vi "RunTest.vi"(8 "error in (no error)":errorcluster, 11 "AjustesPrevios in":refnum<class "AjustesPrevios.lvclass">) -> (0 "error out":errorcluster, 2 "resultado":string, 3 "AjustesPrevios out":refnum<class "AjustesPrevios.lvclass">)   [LabVIEW 2019, in "AjustesPrevios.lvclass"]
uses:
  AjustesPrevios.lvclass
  Prueba04/Control/Slide.ctl
  Controles/MessageAjustesPrev.ctl
  Controles/EstadosAjsutesPrev.ctl
  AjustesPrevios.lvclass/AjustesPrevios.ctl
  QMH/Message Queue/Enqueue Message (Single).vi
  RerenceAllControlsToolkit/_get control reference by name.vi
  RerenceAllControlsToolkit/_get mutiple control reference by name.vi
  Globals/globales.vi
  <vilib>/Utility/miscctls.llb/LVRowAndColumnTypeDef.ctl
  Prueba/Prueba.lvclass
  QMH/User Event - Stop/User Event - Stop.lvlib
  QMH/Message Queue/Message Queue.lvlib
  Prueba04/Prueba04.lvclass
panel:
  out "Sim":bool
  out "Vguardado":dbl
  out "size_frec":i32
  in  "Tabs":enum32{"Ajustes 1", "Ajustes 2", "Ajustes 3"}(tab)
  out "factor_correccion_enviado":dbl format="%#.5g"
  in  "aplicar FC":bool
  out "Voltaje mV":dbl format="%#.3g"
  out "Nivel Medido":dbl format="%#.2g"
  out "temperatura":dbl
  out "presion":dbl
  in  "humedad":dbl
  out "nivel_emitido":dbl
  out "factor_correccion":dbl format="%#.5g"
  in  "siguiente1":bool
  in  "Sensibilidad":dbl(knob)=0.1 scale=0.01..1.0 scale format="%#_6p"
  out "voltaje a CAM":dbl format="%.1f"
  out "frecuencia":dbl
  in  "guardar":bool
  in  "generar":bool
  in  "anterior2":bool
  in  "ajusteAmp(mV)":T1=1.0 caption="Ajuste de amplitud [V]" scale=0.1..1.5
  in  "siguiente2":bool
  in  "generar_CAM":bool
  out "voltaje":dbl format="%_3g"
  out "frecuencia":dbl
  out "NPS":dbl format="%#_4g"
  in  "anterior3":bool
  in  "terminar":bool
  out "Tabla":string[][](table)
  # "Información Pistófono"
  # "Nivel Medido [dB]"
  # "Factor de Corrección Calculado"
  # "Factor de Corrección Enviado"
  # "Voltaje [V]"
  # "Temperatura [°C]"
  # "Presión [hPa]"
  # "Humedad [%]"
  # "Nivel Emitido [dB]"
  # "Ajuste Previo 1 : Igualación de Patrones"
  # "Monitoreo"
  # "Voltaje a CAM"
  # "V"
  # "Frecuencia"
  # "Hz"
  # "Ajuste Previo 2 : Ajuste Acústico Emisor Multitono"
  # "Monitoreo"
  # "NPS"
  # "dB"
  # "Voltaje a CAM"
  # "V"
  # "Frecuencia"
  # "Hz"
  # "Ajuste Previo 3 : Niveles de Presión Sonora de Referencia"
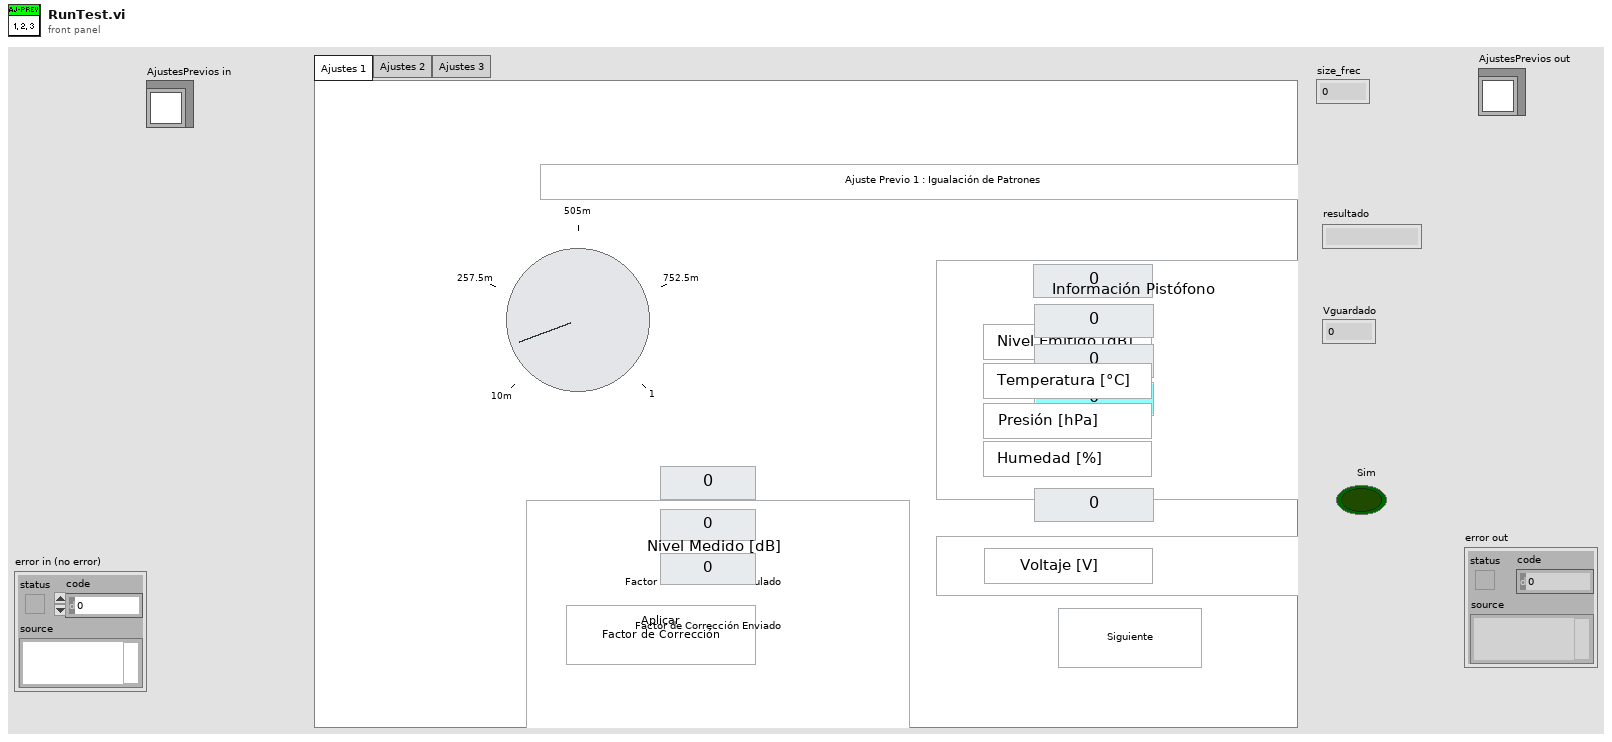
[diagram p1: front panel]
types:
  T1 = typedef "Prueba04.lvclass/Slide.ctl" = dbl
  T2 = typedef "Prueba.lvclass/MessageAjustesPrev.ctl" = cluster{"Estados":T3, "Data":variant}
  T3 = typedef "Prueba.lvclass/EstadosAjsutesPrev.ctl" = enum16{"inicio", "iniciaInstrumentos", "configurarTabla", "Ajustes1", "escribeSensib", "aplicarFC", "escribir_datos_igual_patrones", "preguntar_gen", "Ajustes2", "generar", "detenerGEN", "monitorear", "guardar", "Ajustes3", "generarCAM_94", "avisoParaCAM114", "generarCAM_114", "salir", "error", "reconec_pistofono"}
  T4 = typedef "LVRowAndColumnTypeDef.ctl" = cluster{"Row":i32, "Column":i32}
  T5 = typedef "Message Queue.lvlib/All Message Queues.ctl" = cluster{"MHL":refnum<queue>, "Inst_CNT90":refnum<queue>, "Inst_DS360":refnum<queue>, "Inst_Keithley2002":refnum<queue>, "Inst_DAQ":refnum<queue>, "BD":refnum<queue>, "Pistofono":refnum<queue>, "Nexus":refnum<queue>}
  T6 = enum8{"Enabled", "Disabled", "Disabled and Grayed Out"}
  T7 = cluster{"ControlName":string, "ControlReference":refnum<vi>}[]
  T8 = cluster{"Nivel Emitido Pistófono [dB]":dbl, "Temperatura interna Pistófono[ºC]":dbl, "Presión Medida Pistófono  [hPa]":dbl, "Humedad Relativa Aire [%]":dbl, "FactorCorreccionSensNexus":dbl}
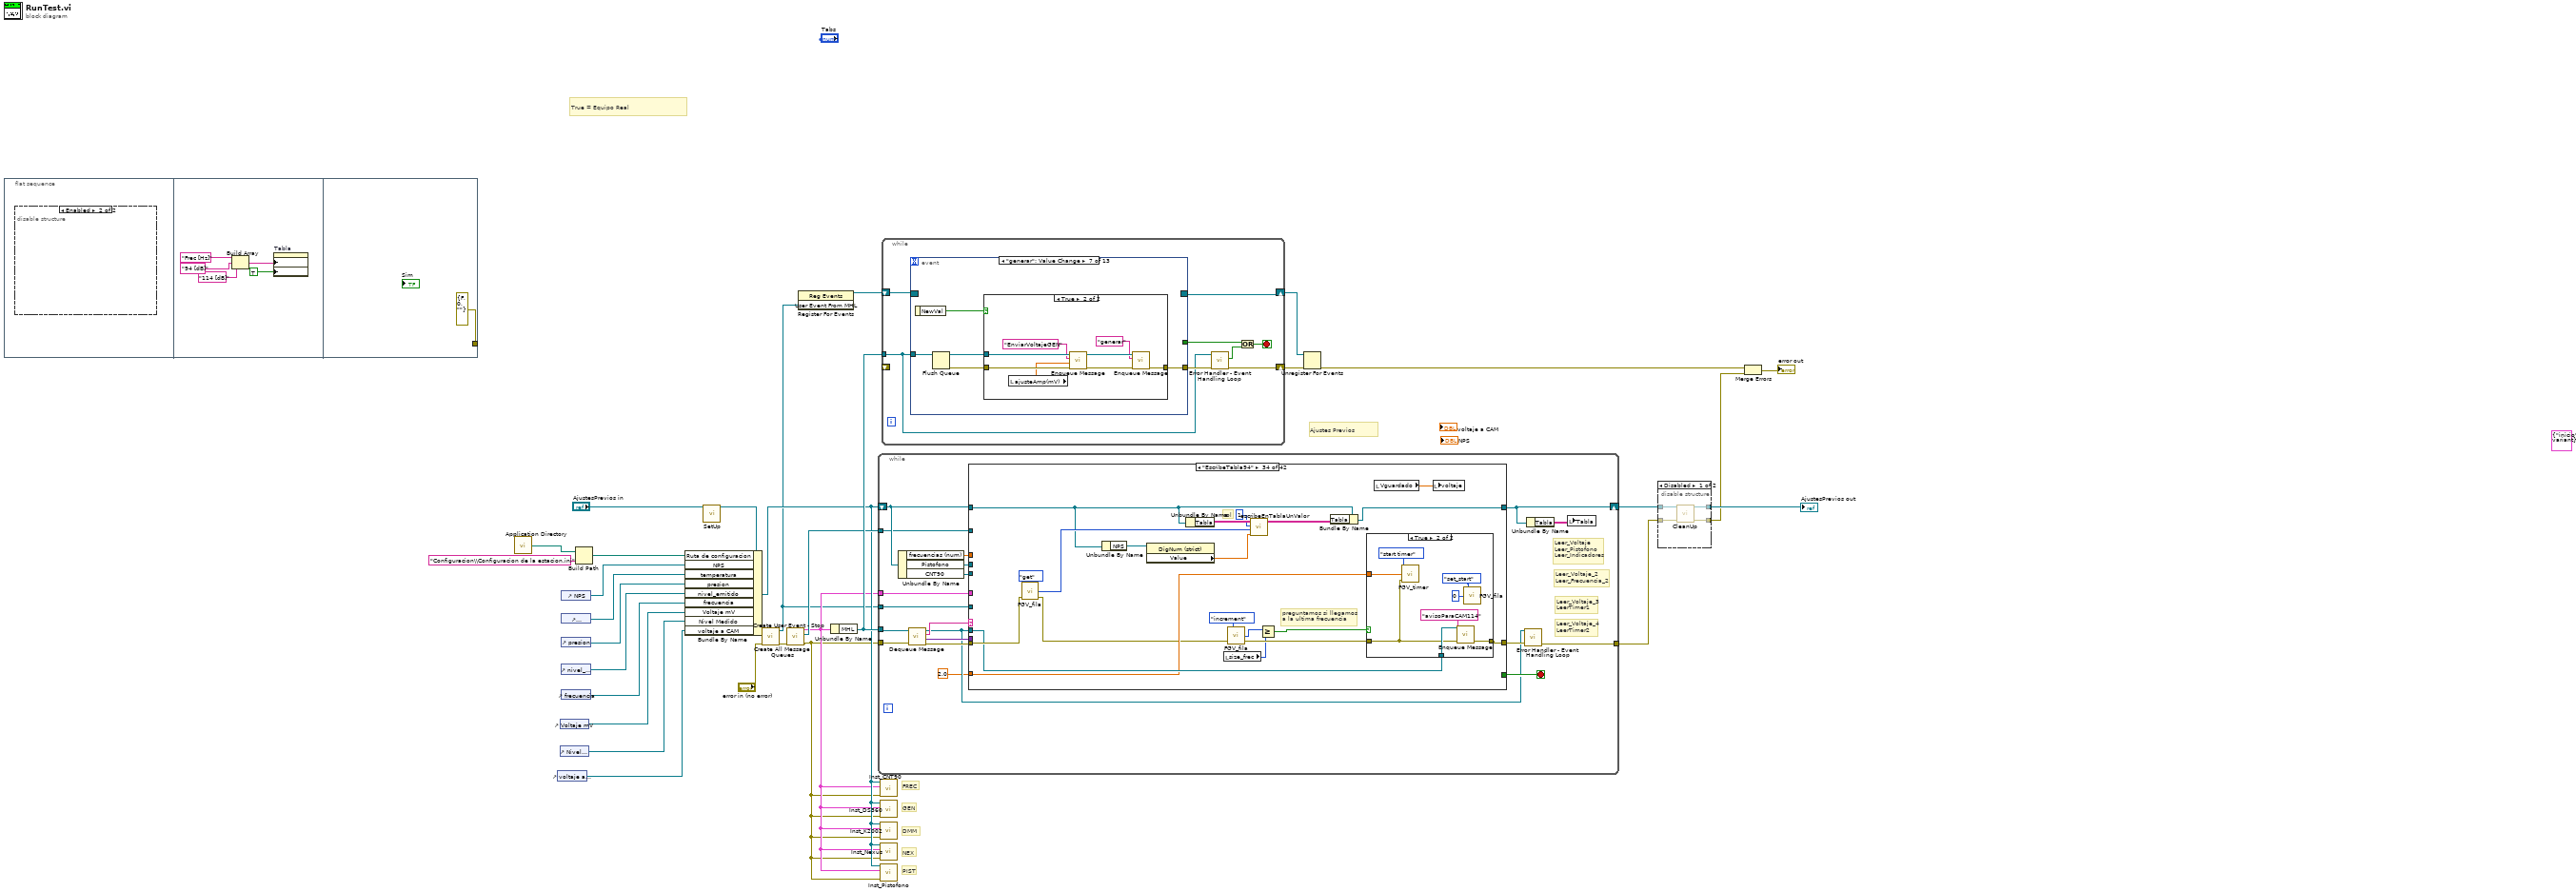
[diagram p0: block diagram]
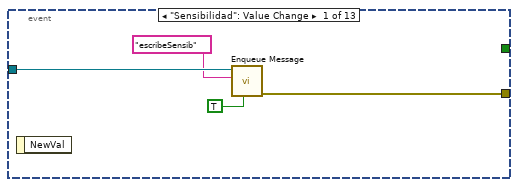
[diagram p3: hidden frame]
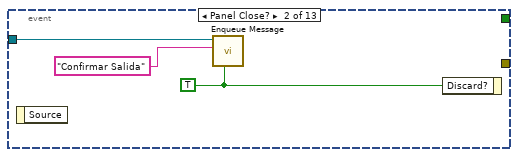
[diagram p4: hidden frame]
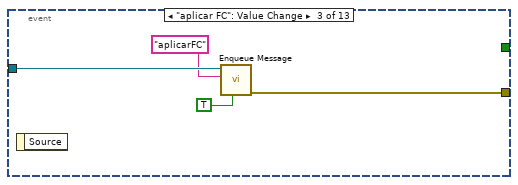
[diagram p5: hidden frame]
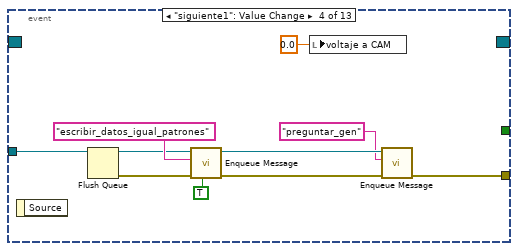
[diagram p6: hidden frame]
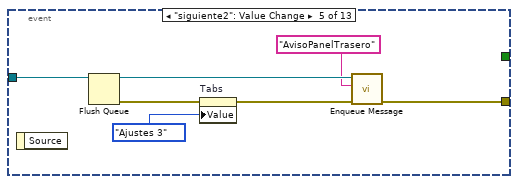
[diagram p7: hidden frame]
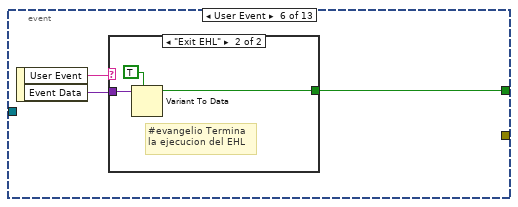
[diagram p8: hidden frame]
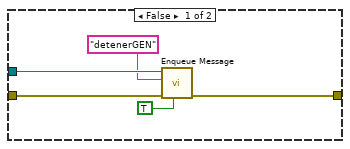
[diagram p10: hidden frame]
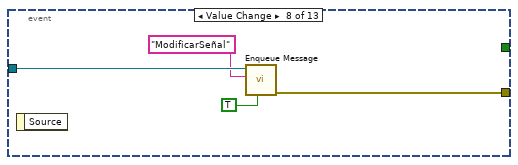
[diagram p11: hidden frame]
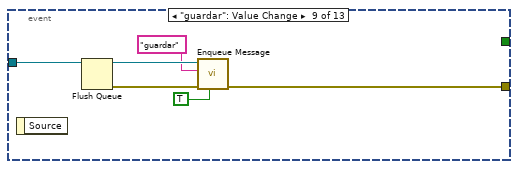
[diagram p12: hidden frame]
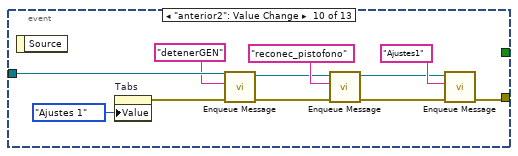
[diagram p13: hidden frame]
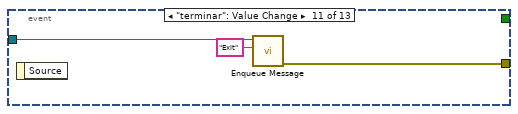
[diagram p14: hidden frame]
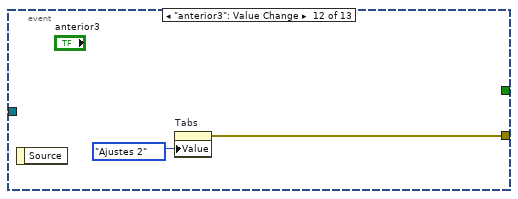
[diagram p15: hidden frame]
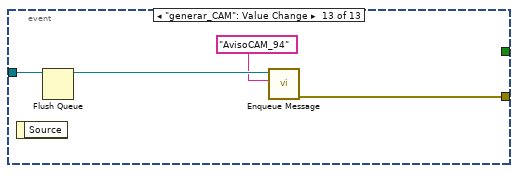
[diagram p16: hidden frame]
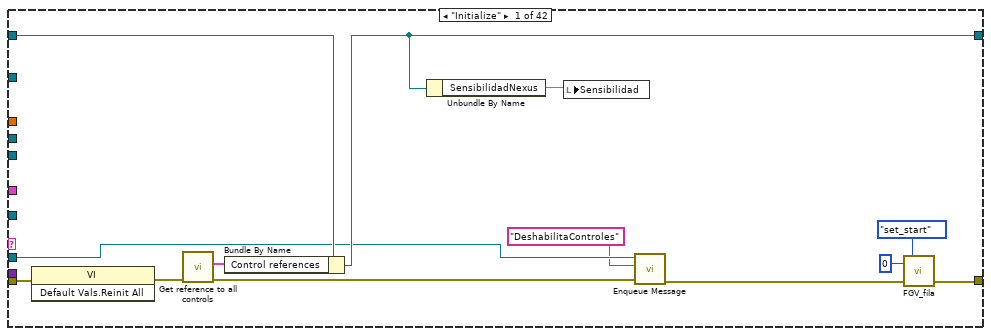
[diagram p17: hidden frame]
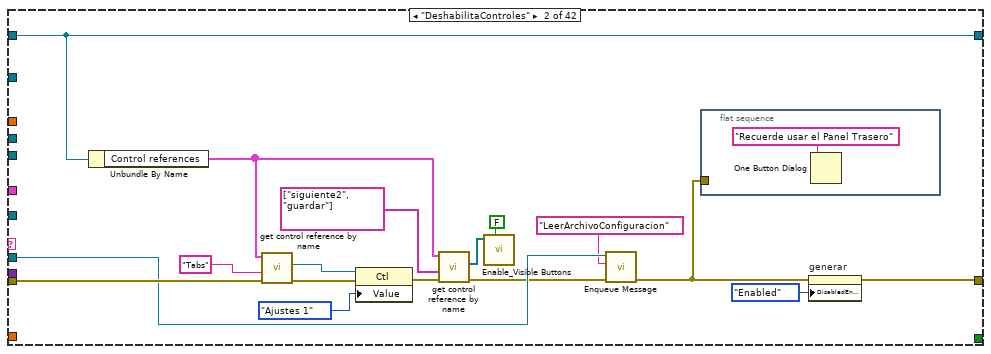
[diagram p18: hidden frame]
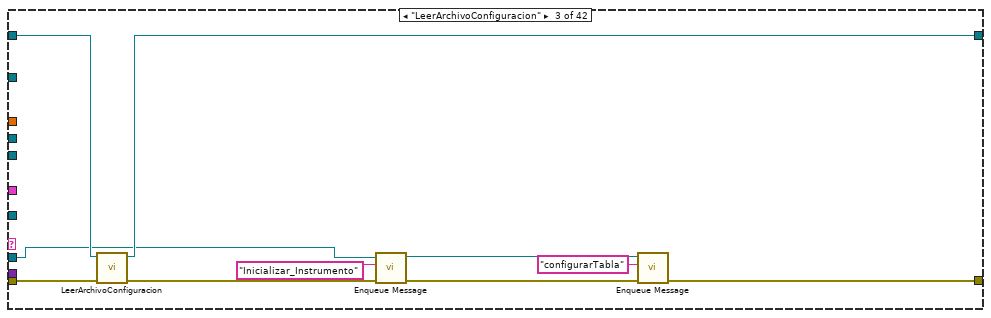
[diagram p19: hidden frame]
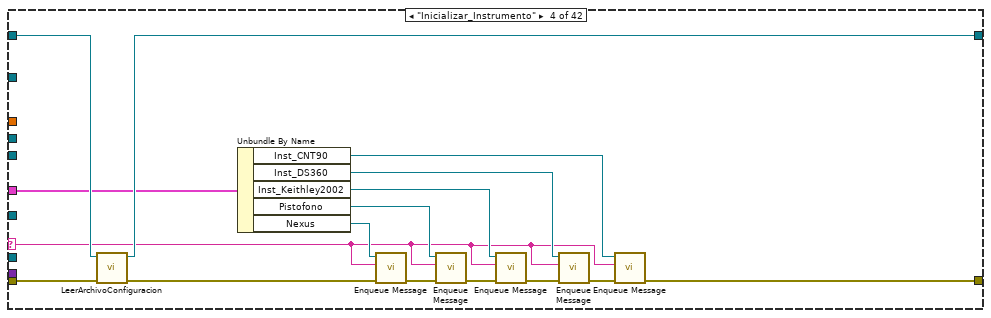
[diagram p20: hidden frame]
diagram:
  (unwired) T2 {"Estados"=enum."inicio", "Data"=variant}
  # "PIST"
  # "NEX"
  # "FREC"
  # "GEN"
  # "DMM"
  # "Ajustes Previos"
  # "True = Equipo Real"
  n1 = flat-sequence {
    tunnel: [errorcluster {"status"=FALSE, "code"=0, "source"=""} ("error in (no error)")] -> _
    frame #0 {
      n2 = disable-structure shown="Enabled" {
        frame Disabled {
          n3 = Bundle By Name(cluster=T4 {"Row"=0, "Column"=0} ("Active Cell:Active Cell"), "Row"=-2, "Column"=-2) -> (w36:T4)
          n4 = property on="Tabla" class="Tbl (strict)"("Active Cell"=w36, "CellFontSize"=u32 20 ("Active Cell:Cell Font:Size"), "Justify"=enum16{"Left", "Center", "Right"}."Center" ("Active Cell:Cell Justification")) -> ()  [unwired: 2 in, 2 out]
        }
        frame Enabled {
        }
      }
    }
    frame #1 {
      n5 = Build Array("Frec [Hz]", "94 [dB]", "114 [dB]" ("element")) -> (w38:string[])
      n6 = property on="Tabla" class="Tbl (strict)"("Column Headers[]"=w38, "Col Headers Vis"=TRUE ("Visible Items:Column Headers Visible")) -> ()  [unwired: 2 in, 2 out]
    }
    frame #2 {
    }
  }
  n7 = call <vilib>:"Application Directory.vi"() -> ("Application Directory"=w20:path)
  n8 = control-ref of="voltaje a CAM"() -> (w1:refnum<vi>)
  n9 = control-ref of="Voltaje mV"() -> (w3:refnum<vi>)
  n10 = control-ref of="Nivel Medido"() -> (w2:refnum<vi>)
  n11 = control-ref of="NPS"() -> (w8:refnum<vi>)
  n12 = control-ref of="temperatura"() -> (w7:refnum<vi>)
  n13 = control-ref of="presion"() -> (w6:refnum<vi>)
  n14 = control-ref of="nivel_emitido"() -> (w5:refnum<vi>)
  n15 = control-ref of="frecuencia"() -> (w4:refnum<vi>)
  n16 = Build Path(base path=w20, name or relative path="Configuracion\\Configuracion de la estacion.ini") -> (appended path=w19:path)
  n17 = call-dynamic "SetUp.vi"("AjustesPrevios in"="AjustesPrevios in") -> ("AjustesPrevios out"=w18:refnum<class "AjustesPrevios.lvclass">)  [unwired: 9 in, 1 out]
  n18 = Bundle By Name(cluster=w18, "Ruta de configuracion"=w19, "NPS"=w8, "temperatura"=w7, "presion"=w6, "nivel_emitido"=w5, "frecuencia"=w4, "Voltaje mV"=w3, "Nivel Medido"=w2, "voltaje a CAM"=w1) -> (w14:refnum<class "AjustesPrevios.lvclass">)
  n19 = call "Create User Event - Stop.vi"("error in (no error)"="error in (no error)") -> ("error out"=w22:errorcluster, "User Event From MHL"=w12:refnum<user-event>)  [unwired: 9 in]
  n20 = call "Create All Message Queues.vi"("error in (no error)"=w22) -> ("error out"=w9:errorcluster, "PL Queues Array"=w15:refnum<queue>[], "All Message Queues out"=w13:T5)  [unwired: 8 in]
  n21 = register-events(w12) -> (reference out=w26:refnum<event-registration>)  [unwired: 2 in, 1 out]
  n22 = Unbundle By Name(w13) -> ("MHL"=w16:refnum<queue>)
  n23 = while {
    tunnel: w16 -> [w54]
    tunnel: w9 -> [w53]
    shift-right: [w59] -> w27
    shift-left: w14 -> [w60]
    tunnel: w13 -> [w49]
    tunnel: w15 -> [w48]
    tunnel: w12 -> [w47]
    tunnel: [w44] -> w11
    stop <- w61 stop-if-true
    # "Leer_Voltaje_4\nLeerTimer2"
    # "Leer_Voltaje_3\nLeerTimer1"
    # "Leer_Voltaje_2\nLeer_Frecuencia_2"
    # "Leer_Voltaje\nLeer_Pistofono\nLeer_Indicadores"
    n24 = Unbundle By Name(w60) -> ("frecuencias (num)"=w56:dbl[], "Pistofono"=w57:refnum<class "Pistofono.lvclass">, "CNT90"=w55:refnum<class "CNT90.lvclass">)
    n25 = call "Dequeue Message.vi"("error in (no error)"=w53, "Message Queue"=w54) -> ("error out"=w52:errorcluster, "Message Data"=w50:variant, "Message"=w51:string, "dup Message Queue"=w45:refnum<queue>)  [unwired: 6 in]
    n26 = case shown="\"EscribeTabla94\"" w51 {
      selector: w51 -> [_ _ _ w103 _ w129 _ _ _ _ _ _ _ _ _ _ _ _ _ _ _ _ _ _ _ _ _ _ _ _ _ _ _ _ _ _ _ _ w570 _ _ _]
      tunnel: w52 -> [w69 w90 w101 w117 w127 w141 w153 w156 w173 w184 w195 w206 w222 w234 w239 w245 w265 w280 w284 w299 w317 w328 w334 w349 w359 w367 w369 w378 w388 w397 w416 w423 w435 w468 w493 w503 w515 w536 w573 w590 w595 w597]
      tunnel: [w74 w76 w97 w102 w121 w128 w143 w155 w173 w174 w185 w196 w210 w229 w238 w247 w266 w280 w281 w295 w307 w318 w330 w344 w350 w365 w369 w378 w385 w396 w405 w421 w441 w466 w487 w498 w513 w545 w566 w584 w595 w597] -> w46
      tunnel: [_ _ _ _ _ _ _ _ _ _ _ _ _ _ _ _ _ _ _ _ _ _ _ _ _ _ _ _ _ _ _ _ _ _ _ _ _ _ w568 _ _ _] -> w61
      tunnel: w60 -> [w67 w91 w99 w115 w124 w140 w152 w162 w172 w183 w194 w205 w217 w232 w243 w250 w259 w279 w293 w306 w316 w327 w340 w345 w358 w366 w368 w377 w382 w398 w418 w432 w450 w453 w492 w512 w529 w532 w569 w593 w594 w596]
      tunnel: [w66 w91 w98 w114 w122 w140 w152 w162 w172 w183 w194 w205 w219 w233 w244 w257 w258 w279 w293 w306 w316 w327 w340 w345 w356 w366 w368 w375 w382 w398 w418 w432 w450 w460 w492 w512 w529 w540 w569 w593 w594 w596] -> w59
      tunnel: w57 -> [_ _ _ _ _ _ _ _ _ _ _ _ _ _ _ _ _ _ _ _ _ _ _ _ _ _ _ _ _ _ _ _ _ _ _ _ _ _ _ _ _ _]
      tunnel: w56 -> [_ _ _ _ _ _ _ _ _ _ _ _ _ _ _ _ _ _ _ _ _ _ _ _ _ _ _ _ _ _ _ _ w436 _ _ _ w517 _ _ _ _ _]
      tunnel: w55 -> [_ _ _ _ _ _ _ _ _ _ _ _ _ _ _ _ _ _ _ _ _ _ _ _ _ _ _ _ _ _ _ _ _ _ _ _ _ _ _ _ _ _]
      tunnel: w45 -> [w65 w80 w96 _ w119 _ _ w157 _ w182 w193 w204 w212 _ _ _ w263 _ _ w296 w315 w326 w333 _ w354 _ _ _ w386 w395 w409 w420 w443 w458 w491 w502 w514 w537 w572 w586 _ _]
      tunnel: w50 -> [_ _ _ _ _ _ _ _ _ _ _ _ _ _ _ _ _ _ w283 _ _ _ _ _ _ _ _ _ _ _ _ _ _ _ _ _ _ _ _ w589 _ _]
      tunnel: w49 -> [_ _ _ w113 _ w139 w151 _ _ w180 w191 w202 _ w228 w242 w249 _ _ w282 w298 w313 w324 w332 w348 _ w364 _ _ w387 _ w415 w422 _ _ _ w501 _ _ _ _ _ _]
      tunnel: w48 -> [_ _ _ _ _ _ _ _ _ _ _ _ _ _ _ _ _ _ _ _ _ _ _ _ _ _ _ _ _ _ _ _ _ _ _ _ _ _ w567 _ _ _]
      tunnel: w47 -> [_ _ _ _ _ _ _ _ _ _ _ _ _ _ _ _ _ _ _ _ _ _ _ _ _ _ _ _ _ _ _ _ _ _ _ _ _ _ w571 _ _ _]
      tunnel: 2.0 ("time target") -> [_ _ _ _ _ _ _ _ _ _ _ _ _ _ _ _ _ _ _ _ _ _ _ _ _ _ _ _ _ _ w402 _ _ w455 w485 _ _ w533 _ _ _ _]
      frame "Initialize" {
        n27 = invoke class="VI" method="Default Vals.Reinit All"(error in=w69) -> (error out=w70:errorcluster)  [unwired: 2 in, 2 out]
        n28 = call "Get reference to all controls.vi"("error in (no error)"=w70) -> ("error out"=w63:errorcluster, "Control references"=w68:T7)  [unwired: 5 in]
        n29 = Bundle By Name(cluster=w67, "Control references"=w68) -> (w66:refnum<class "AjustesPrevios.lvclass">)
        n30 = Unbundle By Name(w66) -> ("SensibilidadNexus"=w71:dbl)
        n31 = local write "Sensibilidad"(w71) -> ()
        n32 = call-poly "Enqueue Message.vi"("error in (no error)"=w63, "Message"="DeshabilitaControles", "Message Queue"=w65) -> ("error out"=w62:errorcluster)  [unwired: 7 in, 1 out]
        n33 = call "FGV_fila.vi"("error in (no error)"=w62, "fila_inicial"=0, "action"=enum16{"increment", "set_start", "get"}."set_start") -> ("error out"=w74:errorcluster)  [unwired: 1 in, 1 out]
      }
      frame "DeshabilitaControles" {
        n34 = Unbundle By Name(w91) -> ("Control references"=w81:T7)
        n35 = call-poly "get control reference by name.vi"("error in (no error)"=w90, "Control name"="Tabs", "Control references"=w81) -> ("error out"=w88:errorcluster, "Ctl Refnum"=w85:refnum<vi>)  [unwired: 3 in]
        n36 = property on="Property Node" class="Ctl"(reference=w85, error in=w88, "Value"=enum32{"Ajustes 1", "Ajustes 2", "Ajustes 3"}."Ajustes 1" ("Tabs")) -> (error out=w87:errorcluster)  [unwired: 1 out]
        n37 = call-poly "get control reference by name.vi"("error in (no error)"=w87, "Control names"=string[] ["siguiente2", "guardar"] ("Control name"), "Control references"=w81) -> ("error out"=w79:errorcluster, "References"=w82:refnum<vi>[])  [unwired: 3 in]
        n38 = call "Enable_Visible Buttons.vi"("Enable? (T)"=FALSE, "Controls Ref Array"=w82) -> ()  [unwired: 10 in]
        n39 = call-poly "Enqueue Message.vi"("error in (no error)"=w79, "Message"="LeerArchivoConfiguracion", "Message Queue"=w80) -> ("error out"=w77:errorcluster)  [unwired: 7 in, 1 out]
        n40 = flat-sequence {
          tunnel: w77 -> [_]
          frame #0 {
            n41 = One Button Dialog(message="Recuerde usar el Panel Trasero") -> ()  [unwired: 1 in, 1 out]
          }
        }
        n42 = property on="generar" class="Bool"(error in=w77, "DisabledEnum"=T6."Enabled" ("Disabled")) -> (error out=w76:errorcluster)  [unwired: 1 in, 1 out]
      }
      frame "LeerArchivoConfiguracion" {
        n43 = call "LeerArchivoConfiguracion.vi"("error in"=w101, "AjustesPrevios in"=w99) -> ("error out"=w100:errorcluster, "AjustesPrevios out"=w98:refnum<class "AjustesPrevios.lvclass">)  [unwired: 8 in]
        n44 = call-poly "Enqueue Message.vi"("error in (no error)"=w100, "Message"="Inicializar_Instrumento", "Message Queue"=w96) -> ("error out"=w97:errorcluster, "dup Message Queue"=w94:refnum<queue>)  [unwired: 7 in]
        n45 = call-poly "Enqueue Message.vi"("Message"="configurarTabla", "Message Queue"=w94) -> ()  [unwired: 8 in, 2 out]
      }
      frame "Inicializar_Instrumento" {
        n46 = call "LeerArchivoConfiguracion.vi"("error in"=w117, "AjustesPrevios in"=w115) -> ("error out"=w116:errorcluster, "AjustesPrevios out"=w114:refnum<class "AjustesPrevios.lvclass">)  [unwired: 8 in]
        n47 = Unbundle By Name(w113) -> ("Inst_CNT90"=w108:refnum<queue>, "Inst_DS360"=w107:refnum<queue>, "Inst_Keithley2002"=w106:refnum<queue>, "Pistofono"=w105:refnum<queue>, "Nexus"=w104:refnum<queue>)
        n48 = call-poly "Enqueue Message.vi"("error in (no error)"=w116, "Message"=w103, "Message Queue"=w104) -> ("error out"=w112:errorcluster)  [unwired: 7 in, 1 out]
        n49 = call-poly "Enqueue Message.vi"("error in (no error)"=w112, "Message"=w103, "Message Queue"=w105) -> ("error out"=w111:errorcluster)  [unwired: 7 in, 1 out]
        n50 = call-poly "Enqueue Message.vi"("error in (no error)"=w111, "Message"=w103, "Message Queue"=w106) -> ("error out"=w110:errorcluster)  [unwired: 7 in, 1 out]
        n51 = call-poly "Enqueue Message.vi"("error in (no error)"=w110, "Message"=w103, "Message Queue"=w107) -> ("error out"=w109:errorcluster)  [unwired: 7 in, 1 out]
        n52 = call-poly "Enqueue Message.vi"("error in (no error)"=w109, "Message"=w103, "Message Queue"=w108) -> ("error out"=w102:errorcluster)  [unwired: 7 in, 1 out]
      }
      frame "configurarTabla" {
        n53 = call-poly "Enqueue Message.vi"("error in (no error)"=w127, "Message"="Ajustes1", "Message Queue"=w119) -> ("error out"=w121:errorcluster)  [unwired: 7 in, 1 out]
        n54 = Unbundle By Name(w124) -> ("Tabla"=w126:string[][], "frecuencias"=w120:string[])
        n55 = call "escribeEnTabla.vi"("parametros"=w120, "col"=0, "tabla in"=w126) -> ("tabla out"=w123:string[][])  [unwired: 8 in]
        n56 = Bundle By Name(cluster=w124, "Tabla"=w123) -> (w122:refnum<class "AjustesPrevios.lvclass">)
      }
      frame "Detener_Instrumento" {
        n57 = Unbundle By Name(w139) -> ("Inst_CNT90"=w134:refnum<queue>, "Inst_DS360"=w133:refnum<queue>, "Inst_Keithley2002"=w132:refnum<queue>, "Pistofono"=w131:refnum<queue>, "Nexus"=w130:refnum<queue>)
        n58 = call-poly "Enqueue Message.vi"("error in (no error)"=w141, "Message"=w129, "Message Queue"=w130) -> ("error out"=w138:errorcluster)  [unwired: 7 in, 1 out]
        n59 = call-poly "Enqueue Message.vi"("error in (no error)"=w138, "Message"=w129, "Message Queue"=w131) -> ("error out"=w137:errorcluster)  [unwired: 7 in, 1 out]
        n60 = call-poly "Enqueue Message.vi"("error in (no error)"=w137, "Message"=w129, "Message Queue"=w132) -> ("error out"=w136:errorcluster)  [unwired: 7 in, 1 out]
        n61 = call-poly "Enqueue Message.vi"("error in (no error)"=w136, "Message"=w129, "Message Queue"=w133) -> ("error out"=w135:errorcluster)  [unwired: 7 in, 1 out]
        n62 = call-poly "Enqueue Message.vi"("error in (no error)"=w135, "Message"=w129, "Message Queue"=w134) -> ("error out"=w128:errorcluster)  [unwired: 7 in, 1 out]
      }
      frame "Detener_Instrumento_Final" {
        w142 = "Detener_Instrumento"
        # "No consideramos el pistofono\nporque ya fue desconectado"
        n63 = Unbundle By Name(w151) -> ("Inst_CNT90"=w147:refnum<queue>, "Inst_DS360"=w146:refnum<queue>, "Inst_Keithley2002"=w145:refnum<queue>, "Nexus"=w144:refnum<queue>)  [unwired: 1 out]
        n64 = call-poly "Enqueue Message.vi"("error in (no error)"=w153, "Message"=w142, "Message Queue"=w144) -> ("error out"=w150:errorcluster)  [unwired: 7 in, 1 out]
        n65 = call-poly "Enqueue Message.vi"("error in (no error)"=w150, "Message"=w142, "Message Queue"=w145) -> ("error out"=w149:errorcluster)  [unwired: 7 in, 1 out]
        n66 = call-poly "Enqueue Message.vi"("error in (no error)"=w149, "Message"=w142, "Message Queue"=w146) -> ("error out"=w148:errorcluster)  [unwired: 7 in, 1 out]
        n67 = call-poly "Enqueue Message.vi"("error in (no error)"=w148, "Message"=w142, "Message Queue"=w147) -> ("error out"=w143:errorcluster)  [unwired: 7 in, 1 out]
      }
      frame "Confirmar Salida" {
        n68 = Two Button Dialog(message="¿Quieres cerrar la aplicación?", 1:"No" ("T button name (\"OK\")"), 2:"Si" ("T button name (\"OK\")")) -> (T button?=w158:bool)
        n69 = case shown="True" w158 {
          tunnel: w156 -> [w163 w171]
          tunnel: [w163 w166] -> w155
          tunnel: w157 -> [_ w169]
          tunnel: "Detener_Instrumento" ("Message") -> [_ w167]
          frame False {
          }
          frame True {
            n70 = call-poly "Enqueue Message.vi"("Priority Message? (F)"=TRUE, "error in (no error)"=w171, "Message"=w167, "Message Queue"=w169) -> ("error out"=w170:errorcluster, "dup Message Queue"=w165:refnum<queue>)  [unwired: 6 in]
            n71 = call-poly "Enqueue Message.vi"("error in (no error)"=w170, "Message"="Exit", "Message Queue"=w165) -> ("error out"=w166:errorcluster)  [unwired: 7 in, 1 out]
          }
        }
      }
      frame "--------------------------Ajustes 1---------------------------" {
      }
      frame "Ajustes1" {
        n72 = Unbundle By Name(w180) -> ("Inst_Keithley2002"=w178:refnum<queue>)
        n73 = call-poly "Enqueue Message.vi"("error in (no error)"=w184, "Message"="Leer_Voltaje", "Message Queue"=w182) -> ("error out"=w177:errorcluster)  [unwired: 7 in, 1 out]
        n74 = call-poly "Enqueue Message.vi"("error in (no error)"=w177, "Message"="Leer_Instrumento", "Message Queue"=w178) -> ("error out"=w175:errorcluster)  [unwired: 7 in, 1 out]
        n75 = call "Time Delay2"("error in (no error)"=w175, "Delay Time (s)"=1.0) -> ("error out"=w174:errorcluster)  [unwired: 9 in]
      }
      frame "Leer_Voltaje" {
        n76 = Unbundle By Name(w191) -> ("Inst_Keithley2002"=w189:refnum<queue>)
        n77 = call-poly "Enqueue Message.vi"("error in (no error)"=w195, "Message"="Leer_Pistofono", "Message Queue"=w193) -> ("error out"=w188:errorcluster)  [unwired: 7 in, 1 out]
        n78 = call-poly "Enqueue Message.vi"("error in (no error)"=w188, "Message"="Leer_Instrumento", "Message Queue"=w189) -> ("error out"=w186:errorcluster)  [unwired: 7 in, 1 out]
        n79 = call "Time Delay3"("error in (no error)"=w186, "Delay Time (s)"=1.0) -> ("error out"=w185:errorcluster)  [unwired: 9 in]
      }
      frame "Leer_Pistofono" {
        n80 = Unbundle By Name(w202) -> ("Pistofono"=w200:refnum<queue>)
        n81 = call-poly "Enqueue Message.vi"("error in (no error)"=w206, "Message"="Leer_Indicadores", "Message Queue"=w204) -> ("error out"=w199:errorcluster)  [unwired: 7 in, 1 out]
        n82 = call-poly "Enqueue Message.vi"("error in (no error)"=w199, "Message"="Leer_Instrumento", "Message Queue"=w200) -> ("error out"=w197:errorcluster)  [unwired: 7 in, 1 out]
        n83 = call "Time Delay4"("error in (no error)"=w197, "Delay Time (s)"=1.0) -> ("error out"=w196:errorcluster)  [unwired: 9 in]
      }
      frame "Leer_Indicadores" {
        n84 = Unbundle By Name(w217) -> ("Voltaje mV"=w216:refnum<vi>, "Nivel Medido"=w215:refnum<vi>, "nivel_emitido"=w209:refnum<vi>)
        n85 = property class="DigNum (strict)"(reference=w209) -> ("Value"=w208:dbl)  [unwired: 1 in, 2 out]
        n86 = property class="DigNum (strict)"(reference=w216) -> ("Value"=w214:dbl)  [unwired: 1 in, 2 out]
        n87 = property class="DigNum (strict)"(reference=w215) -> ("Value"=w207:dbl)  [unwired: 1 in, 2 out]
        n88 = call-poly "Enqueue Message.vi"("error in (no error)"=w222, "Message"="Leer_Voltaje", "Message Queue"=w212) -> ("error out"=w213:errorcluster)  [unwired: 7 in, 1 out]
        n89 = disable-structure shown="Disabled" {
          frame Disabled {
            n90 = local read "nivel_emitido"() -> ()  [unwired: 1 out]
          }
          frame Enabled {
          }
        }
        n91 = call "FactorCorreccion.vi"("error in (no error)"=w213, "Nivel Medido"=w207, "Nivel Emitido"=w208) -> ("error out"=w221:errorcluster, "factor_correccion"=→"factor_correccion":dbl)  [unwired: 7 in]
        n92 = call "Time Delay17"("error in (no error)"=w221) -> ("error out"=w210:errorcluster)  [unwired: 10 in]
        n93 = Bundle By Name(cluster=w217, "Voltaje enviado a CAM"=w214, "Humedad"="humedad") -> (w219:refnum<class "AjustesPrevios.lvclass">)
      }
      frame "aplicarFC" {
        n94 = Unbundle By Name(w228) -> ("Nexus"=w227:refnum<queue>)
        n95 = call "Time Delay6"("error in (no error)"=w234, "Delay Time (s)"=1.0) -> ("error out"=w224:errorcluster)  [unwired: 9 in]
        n96 = local read "factor_correccion"() -> (w226:dbl)
        "factor_correccion_enviado" <- w226
        n97 = Unbundle By Name(w232) -> ("igualacion_de_patrones"=w231:T8)
        n98 = Bundle By Name(cluster=w231, "FactorCorreccionSensNexus"=w226) -> (w230:T8)
        n99 = call-poly "Enqueue Message.vi"("error in (no error)"=w224, "Message Data"=w226, "Message"="AplicarFactorCorreccion", "Message Queue"=w227) -> ("error out"=w229:errorcluster)  [unwired: 6 in, 1 out]
        n100 = Bundle By Name(cluster=w232, "igualacion_de_patrones"=w230) -> (w233:refnum<class "AjustesPrevios.lvclass">)
      }
      frame "escribeSensib" {
        n101 = local read "Sensibilidad"() -> (w237:dbl)
        n102 = Unbundle By Name(w242) -> ("Nexus"=w241:refnum<queue>)
        n103 = call "Time Delay5"("error in (no error)"=w239, "Delay Time (s)"=1.0) -> ("error out"=w236:errorcluster)  [unwired: 9 in]
        n104 = call-poly "Enqueue Message.vi"("error in (no error)"=w236, "Message Data"=w237, "Message"="EscribirSensibilidad", "Message Queue"=w241) -> ("error out"=w238:errorcluster)  [unwired: 6 in, 1 out]
        n105 = Bundle By Name(cluster=w243, "SensibilidadNexus"=w237) -> (w244:refnum<class "AjustesPrevios.lvclass">)
      }
      frame "escribir_datos_igual_patrones" {
        n106 = Unbundle By Name(w249) -> ("Pistofono"=w248:refnum<queue>)
        n107 = call-poly "Enqueue Message.vi"("error in (no error)"=w245, "Message"="Detener_Instrumento", "Message Queue"=w248) -> ("error out"=w247:errorcluster)  [unwired: 7 in, 1 out]
        n108 = Unbundle By Name(w250) -> ("igualacion_de_patrones"=w256:T8)
        n109 = local read "nivel_emitido"() -> (w255:dbl)
        n110 = local read "temperatura"() -> (w254:dbl)
        n111 = local read "humedad"() -> (w252:dbl)
        n112 = local read "presion"() -> (w253:dbl)
        n113 = Bundle By Name(cluster=w256, "Nivel Emitido Pistófono [dB]"=w255, "Temperatura interna Pistófono[ºC]"=w254, "Presión Medida Pistófono  [hPa]"=w253, "Humedad Relativa Aire [%]"=w252) -> (w251:T8)
        n114 = Bundle By Name(cluster=w250, "igualacion_de_patrones"=w251) -> (w257:refnum<class "AjustesPrevios.lvclass">)
      }
      frame "preguntar_gen" {
        # "Escribe en Archivo INI"
        n115 = call "selccionaGenerador.vi"("error in (no error)"=w265) -> ("error out"=w264:errorcluster, "Generador"=w261:string)  [unwired: 1 in]
        n116 = call "EscribirArchivoConfiguracion.vi"("error in"=w264, "TipoGenerador"=w261, "AjustesPrevios in"=w259) -> ("error out"=w262:errorcluster, "TipoGenerador out"=w260:string, "AjustesPrevios out"=w258:refnum<class "AjustesPrevios.lvclass">)  [unwired: 6 in]
        n117 = case shown="\"Externo\", Default" w260 {
          tunnel: [w268 w274] -> w266
          tunnel: w262 -> [w272 w275]
          tunnel: w263 -> [w273 _]
          frame "Interno" {
            n118 = call-poly "Enqueue Message.vi"("error in (no error)"=w272, "Message"="Detener_Instrumento", "Message Queue"=w273) -> ("error out"=w269:errorcluster, "dup Message Queue"=w270:refnum<queue>)  [unwired: 7 in]
            n119 = call-poly "Enqueue Message.vi"("error in (no error)"=w269, "Message"="Exit", "Message Queue"=w270) -> ("error out"=w268:errorcluster)  [unwired: 7 in, 1 out]
          }
          frame "Externo", Default {
            n120 = local read "ajusteAmp(mV)"() -> (w277:T1)
            n121 = property on="Tabs" class="TabCtl (strict)"(error in=w275, "Value"=enum32{"Ajustes 1", "Ajustes 2", "Ajustes 3"}."Ajustes 2" ("Tabs")) -> (error out=w274:errorcluster)  [unwired: 1 in, 1 out]
            n122 = One Button Dialog(message="Recuerde usar el Panel Delantero") -> ()  [unwired: 1 in, 1 out]
            n123 = local write "voltaje a CAM"(w277) -> ()
          }
        }
      }
      frame "--------------------------Ajustes 2---------------------------" {
      }
      frame "EnviarVoltajeGEN" {
        n124 = Unbundle By Name(w282) -> ("Inst_DS360"=w287:refnum<queue>, "Inst_Keithley2002"=w292:refnum<queue>)
        n125 = Variant To Data(error in=w284, type=0.0, Variant=w283) -> (data=w285:dbl, error out=w290:errorcluster)
        n126 = call-poly "Enqueue Message.vi"("error in (no error)"=w290, "Message Data"=w285, "Message"="ActualizarVoltaje", "Message Queue"=w292) -> ("error out"=w288:errorcluster)  [unwired: 6 in, 1 out]
        n127 = call-poly "Enqueue Message.vi"("error in (no error)"=w288, "Message Data"=w285, "Message"="GenerarSeñal", "Message Queue"=w287) -> ("error out"=w281:errorcluster)  [unwired: 6 in, 1 out]
      }
      frame "generar" {
        n128 = Unbundle By Name(w298) -> ("Inst_DS360"=w304:refnum<queue>)
        n129 = call-poly "Enqueue Message.vi"("error in (no error)"=w299, "Message"="Habilitar_Generador", "Message Queue"=w304) -> ("error out"=w302:errorcluster)  [unwired: 7 in, 1 out]
        n130 = call "Time Delay7"("error in (no error)"=w302, "Delay Time (s)"=0.5) -> ("error out"=w301:errorcluster)  [unwired: 9 in]
        n131 = call-poly "Enqueue Message.vi"("error in (no error)"=w301, "Message"="Leer_Voltaje_2", "Message Queue"=w296) -> ("error out"=w297:errorcluster)  [unwired: 7 in, 1 out]
        n132 = property on="guardar" class="Bool"(error in=w297, "DisabledEnum"=T6."Enabled" ("Disabled")) -> (error out=w295:errorcluster)  [unwired: 1 in, 1 out]
      }
      frame "Leer_Voltaje_2" {
        n133 = Unbundle By Name(w313) -> ("Inst_Keithley2002"=w311:refnum<queue>)
        n134 = call-poly "Enqueue Message.vi"("error in (no error)"=w317, "Message"="Leer_Frecuencia_2", "Message Queue"=w315) -> ("error out"=w310:errorcluster)  [unwired: 7 in, 1 out]
        n135 = call-poly "Enqueue Message.vi"("error in (no error)"=w310, "Message"="Leer_Instrumento", "Message Queue"=w311) -> ("error out"=w308:errorcluster)  [unwired: 7 in, 1 out]
        n136 = call "Time Delay8"("error in (no error)"=w308, "Delay Time (s)"=1.0) -> ("error out"=w307:errorcluster)  [unwired: 9 in]
      }
      frame "Leer_Frecuencia_2" {
        n137 = Unbundle By Name(w324) -> ("Inst_CNT90"=w322:refnum<queue>)
        n138 = call-poly "Enqueue Message.vi"("error in (no error)"=w328, "Message"="Leer_Voltaje_2", "Message Queue"=w326) -> ("error out"=w321:errorcluster)  [unwired: 7 in, 1 out]
        n139 = call-poly "Enqueue Message.vi"("error in (no error)"=w321, "Message"="Leer_Instrumento", "Message Queue"=w322) -> ("error out"=w319:errorcluster)  [unwired: 7 in, 1 out]
        n140 = call "Time Delay9"("error in (no error)"=w319, "Delay Time (s)"=1.0) -> ("error out"=w318:errorcluster)  [unwired: 9 in]
      }
      frame "detenerGEN" {
        n141 = Flush Queue(queue=w333, error in (no error)=w334) -> (error out=w336:errorcluster)  [unwired: 2 out]
        n142 = Unbundle By Name(w332) -> ("Inst_DS360"=w338:refnum<queue>)
        n143 = call "Time Delay10"("error in (no error)"=w336, "Delay Time (s)"=0.5) -> ("error out"=w335:errorcluster)  [unwired: 9 in]
        n144 = call-poly "Enqueue Message.vi"("error in (no error)"=w335, "Message"="Deshabilitar_Generador", "Message Queue"=w338) -> ("error out"=w331:errorcluster)  [unwired: 7 in, 1 out]
        n145 = property on="anterior3" class="Bool"(error in=w331, "DisabledEnum"=T6."Enabled" ("Disabled")) -> (error out=w330:errorcluster)  [unwired: 1 in, 1 out]
      }
      frame "ModificarSeñal" {
        n146 = call "Time Delay11"("error in (no error)"=w349, "Delay Time (s)"=1.0) -> ("error out"=w342:errorcluster)  [unwired: 9 in]
        n147 = local read "ajusteAmp(mV)"() -> (w346:T1)
        n148 = Unbundle By Name(w348) -> ("Inst_DS360"=w347:refnum<queue>)
        n149 = call-poly "Enqueue Message.vi"("error in (no error)"=w342, "Message Data"=w346, "Message"="GenerarSeñal", "Message Queue"=w347) -> ("error out"=w344:errorcluster)  [unwired: 6 in, 1 out]
      }
      frame "guardar" {
        n150 = call-poly "Enqueue Message.vi"("error in (no error)"=w359, "Message"="detenerGEN", "Message Queue"=w354) -> ("error out"=w352:errorcluster)  [unwired: 7 in, 1 out]
        n151 = property on="siguiente2" class="Bool"(error in=w352, "DisabledEnum"=T6."Enabled" ("Disabled")) -> (error out=w351:errorcluster)  [unwired: 1 in, 1 out]
        n152 = local read "voltaje a CAM"() -> (w355:dbl)
        "Vguardado" <- w355
        n153 = flat-sequence {
          tunnel: [w360] -> w350
          tunnel: w351 -> [w360]
          frame #0 {
            n154 = One Button Dialog(message="Voltaje guardado") -> ()  [unwired: 1 in, 1 out]
          }
        }
        n155 = Bundle By Name(cluster=w358, "Voltaje enviado a CAM"=w355) -> (w356:refnum<class "AjustesPrevios.lvclass">)
        n156 = global write "globales.vi" "Vguardado"(w355) -> ()
      }
      frame "reconec_pistofono" {
        n157 = Unbundle By Name(w364) -> ("Pistofono"=w363:refnum<queue>)
        n158 = call-poly "Enqueue Message.vi"("error in (no error)"=w367, "Message"="Inicializar_Instrumento", "Message Queue"=w363) -> ("error out"=w365:errorcluster)  [unwired: 7 in, 1 out]
      }
      frame "--------------------------Ajustes 3---------------------------" {
      }
      frame "AvisoPanelTrasero" {
        w370 = string[] ["--", "--", "--", "--", "--", "--", "---", "--", "--", "--", "--"] ("new element/subarray")
        n159 = One Button Dialog(message="Recuerde usar el Panel Trasero") -> ()  [unwired: 1 in, 1 out]
        n160 = local write "NPS"(0.0 ("NPS")) -> ()
        n161 = Unbundle By Name(w377) -> ("Tabla"=w376:string[][])
        n162 = Replace Array Subset(array=w376, new element=w370, index (col)=1 ("disabled index (col)")) -> (w373:string[][])  [unwired: 1 in]
        n163 = Replace Array Subset(array=w373, new element=w370, index (col)=2 ("disabled index (col)")) -> (w372:string[][])  [unwired: 1 in]
        n164 = Bundle By Name(cluster=w377, "Tabla"=w372) -> (w375:refnum<class "AjustesPrevios.lvclass">)
      }
      frame "generarCAM" {
        n165 = Unbundle By Name(w387) -> ("Inst_DS360"=w384:refnum<queue>)
        n166 = Unbundle By Name(w382) -> ("Voltaje enviado a CAM"=w381:dbl)
        n167 = call-poly "Enqueue Message.vi"("Message Data"=w381, "Message"="GenerarSeñal", "Message Queue"=w384) -> ()  [unwired: 7 in, 2 out]
        n168 = call-poly "Enqueue Message.vi"("error in (no error)"=w388, "Message"="Habilitar_Generador", "Message Queue"=w384) -> ("error out"=w391:errorcluster)  [unwired: 7 in, 1 out]
        n169 = call "Time Delay12"("error in (no error)"=w391, "Delay Time (s)"=1.0) -> ("error out"=w390:errorcluster)  [unwired: 9 in]
        n170 = call-poly "Enqueue Message.vi"("error in (no error)"=w390, "Message"="Leer_Voltaje_3", "Message Queue"=w386) -> ("error out"=w385:errorcluster)  [unwired: 7 in, 1 out]
      }
      frame "AvisoCAM_94" {
        n171 = call-poly "Enqueue Message.vi"("error in (no error)"=w397, "Message"="ActivarGEN_94", "Message Queue"=w395) -> ("error out"=w396:errorcluster)  [unwired: 7 in, 1 out]
        n172 = flat-sequence {
          tunnel: w396 -> [_]
          frame #0 {
            n173 = local write "generar_CAM"(FALSE ("generar_CAM")) -> ()
          }
          frame #1 {
            n174 = One Button Dialog(message="Lleve el CAM a 94 dB") -> ()  [unwired: 1 in, 1 out]
          }
        }
      }
      frame "ActivarGEN_94" {
        # "Inici el Timer"
        # "Envía set point a generador"
        n175 = Unbundle By Name(w415) -> ("Inst_DS360"=w417:refnum<queue>)
        n176 = local read "Vguardado"() -> (w413:dbl)
        n177 = call-poly "Enqueue Message.vi"("error in (no error)"=w416, "Message Data"=w413, "Message"="GenerarSeñal", "Message Queue"=w417) -> ("error out"=w412:errorcluster, "dup Message Queue"=w411:refnum<queue>)  [unwired: 6 in]
        n178 = call-poly "Enqueue Message.vi"("error in (no error)"=w412, "Message"="Habilitar_Generador", "Message Queue"=w411) -> ("error out"=w408:errorcluster)  [unwired: 7 in, 1 out]
        n179 = call-poly "Enqueue Message.vi"("error in (no error)"=w408, "Message"="Leer_Voltaje_3", "Message Queue"=w409) -> ("error out"=w406:errorcluster)  [unwired: 7 in, 1 out]
        n180 = call "FGV_timer.vi"("error in (no error)"=w406, "time target"=w402, "action"=enum16{"get time", "start timer"}."start timer") -> ("error out"=w403:errorcluster)  [unwired: 2 out]
        n181 = call "Time Delay14"("error in (no error)"=w403, "Delay Time (s)"=1.0) -> ("error out"=w405:errorcluster)  [unwired: 9 in]
      }
      frame "Leer_Voltaje_3" {
        n182 = Flush Queue(queue=w420, error in (no error)=w423) -> (queue out=w424:refnum<queue>, error out=w425:errorcluster)  [unwired: 1 out]
        n183 = Unbundle By Name(w422) -> ("Inst_Keithley2002"=w428:refnum<queue>)
        n184 = call-poly "Enqueue Message.vi"("error in (no error)"=w425, "Message"="LeerTimer1", "Message Queue"=w424) -> ("error out"=w431:errorcluster)  [unwired: 7 in, 1 out]
        n185 = local write "generar_CAM"(TRUE ("generar_CAM")) -> ()
        n186 = call-poly "Enqueue Message.vi"("error in (no error)"=w431, "Message"="Leer_Instrumento", "Message Queue"=w428) -> ("error out"=w429:errorcluster)  [unwired: 7 in, 1 out]
        n187 = call "Time Delay15"("error in (no error)"=w429, "Delay Time (s)"=1.0) -> ("error out"=w421:errorcluster)  [unwired: 9 in]
      }
      frame "LeerTimer1" {
        # "si se cumple el timpo nos vamos\na escribir en la tabla, si no, seguimos leyendo\nel voltaje"
        n188 = call "FGV_fila.vi"("error in (no error)"=w435, "action"=enum16{"increment", "set_start", "get"}."get") -> ("error out"=w434:errorcluster, "fila out"=w439:i32)  [unwired: 2 in]
        n189 = Array Size(array=w436) -> (size(s)=→"size_frec":i32)
        n190 = Index Array(array=w436, index=w439) -> (element=w438:dbl)
        n191 = local write "frecuencia"(w438) -> ()
        n192 = call "FGV_timer.vi"("error in (no error)"=w434, "action"=enum16{"get time", "start timer"}."get time") -> ("error out"=w449:errorcluster, "time elapsed?"=w446:bool)  [unwired: 1 in, 1 out]
        n193 = Select(t="EscribeTabla94", s=w446, f="Leer_Voltaje_3") -> (s? t:f=w444:string)
        n194 = call-poly "Enqueue Message.vi"("error in (no error)"=w449, "Message"=w444, "Message Queue"=w443) -> ("error out"=w447:errorcluster)  [unwired: 7 in, 1 out]
        n195 = call "Time Delay"("error in (no error)"=w447, "Delay Time (s)"=1.0) -> ("error out"=w441:errorcluster)  [unwired: 9 in]
      }
      frame "EscribeTabla94" {
        # "preguntamos si llegamos\na la ultima frecuencia"
        # "col"
        n196 = call "FGV_fila.vi"("error in (no error)"=w468, "action"=enum16{"increment", "set_start", "get"}."get") -> ("error out"=w454:errorcluster, "fila out"=w462:i32)  [unwired: 2 in]
        n197 = Unbundle By Name(w453) -> ("NPS"=w452:refnum<vi>)
        n198 = property class="DigNum (strict)"(reference=w452) -> ("Value"=w451:dbl)  [unwired: 1 in, 2 out]
        n199 = Unbundle By Name(w453) -> ("Tabla"=w457:string[][])
        n200 = local read "size_frec"() -> (w463:i32)
        n201 = call "FGV_fila.vi"("error in (no error)"=w454, "action"=enum16{"increment", "set_start", "get"}."increment") -> ("error out"=w467:errorcluster, "fila out"=w464:i32)  [unwired: 2 in]
        n202 = call "escribeEnTablaUnValor.vi"("element"=w451, "fila"=w462, "col"=1, "tabla in"=w457) -> ("tabla out"=w461:string[][])  [unwired: 7 in]
        n203 = Greater Or Equal?(x=w464, y=w463) -> (x >= y?=w465:bool)
        n204 = Bundle By Name(cluster=w453, "Tabla"=w461) -> (w460:refnum<class "AjustesPrevios.lvclass">)
        n205 = case shown="True" w465 {
          tunnel: w467 -> [w473 w477]
          tunnel: [w476 w484] -> w466
          tunnel: w458 -> [w474 w480]
          tunnel: w455 -> [w471 w478]
          frame False {
            n206 = call "FGV_timer.vi"("error in (no error)"=w473, "time target"=w471, "action"=enum16{"get time", "start timer"}."start timer") -> ()  [unwired: 3 out]
            n207 = call-poly "Enqueue Message.vi"("error in (no error)"=w473, "Message"="Leer_Voltaje_3", "Message Queue"=w474) -> ("error out"=w476:errorcluster)  [unwired: 7 in, 1 out]
          }
          frame True {
            n208 = call "FGV_timer.vi"("error in (no error)"=w477, "time target"=w478, "action"=enum16{"get time", "start timer"}."start timer") -> ()  [unwired: 3 out]
            n209 = call-poly "Enqueue Message.vi"("error in (no error)"=w477, "Message"="avisoParaCAM114", "Message Queue"=w480) -> ("error out"=w484:errorcluster)  [unwired: 7 in, 1 out]
            n210 = call "FGV_fila.vi"("fila_inicial"=0, "action"=enum16{"increment", "set_start", "get"}."set_start") -> ()  [unwired: 2 in, 2 out]
          }
        }
        n211 = local read "Vguardado"() -> (w459:dbl)
        n212 = local write "voltaje"(w459) -> ()
      }
      frame "avisoParaCAM114" {
        # "iniciamos timer"
        n213 = call-poly "Enqueue Message.vi"("error in (no error)"=w493, "Message"="Leer_Voltaje_4", "Message Queue"=w491) -> ("error out"=w489:errorcluster)  [unwired: 7 in, 1 out]
        n214 = flat-sequence {
          tunnel: w489 -> [w494]
          tunnel: [w494] -> w488
          frame #0 {
            n215 = local write "generar_CAM"(FALSE ("generar_CAM")) -> ()
            n216 = One Button Dialog(message="Lleve el CAM a 114 dB") -> ()  [unwired: 1 in, 1 out]
          }
        }
        n217 = call "FGV_timer.vi"("error in (no error)"=w488, "time target"=w485, "action"=enum16{"get time", "start timer"}."start timer") -> ("error out"=w487:errorcluster)  [unwired: 2 out]
      }
      frame "Leer_Voltaje_4" {
        n218 = Flush Queue(queue=w502, error in (no error)=w503) -> (queue out=w504:refnum<queue>, error out=w505:errorcluster)  [unwired: 1 out]
        n219 = Unbundle By Name(w501) -> ("Inst_Keithley2002"=w508:refnum<queue>)
        n220 = call-poly "Enqueue Message.vi"("error in (no error)"=w505, "Message"="LeerTimer2", "Message Queue"=w504) -> ("error out"=w511:errorcluster)  [unwired: 7 in, 1 out]
        n221 = local write "generar_CAM"(TRUE ("generar_CAM")) -> ()
        n222 = call-poly "Enqueue Message.vi"("error in (no error)"=w511, "Message"="Leer_Instrumento", "Message Queue"=w508) -> ("error out"=w509:errorcluster)  [unwired: 7 in, 1 out]
        n223 = call "Time Delay13"("error in (no error)"=w509, "Delay Time (s)"=1.0) -> ("error out"=w500:errorcluster)  [unwired: 9 in]
        n224 = property on="anterior3" class="Bool"(error in=w500, "DisabledEnum"=T6."Disabled and Grayed Out" ("Disabled")) -> (error out=w498:errorcluster)  [unwired: 1 in, 1 out]
      }
      frame "LeerTimer2" {
        # "si se cumple el timpo nos vamos\na escribir en la tabla, si no, seguimos leyendo\nel voltaje"
        n225 = call "FGV_fila.vi"("error in (no error)"=w515, "action"=enum16{"increment", "set_start", "get"}."get") -> ("error out"=w518:errorcluster, "fila out"=w520:i32)  [unwired: 2 in]
        n226 = Index Array(array=w517, index=w520) -> (element=w516:dbl)
        n227 = local write "frecuencia"(w516) -> ()
        n228 = call "FGV_timer.vi"("error in (no error)"=w518, "action"=enum16{"get time", "start timer"}."get time") -> ("error out"=w528:errorcluster, "time elapsed?"=w525:bool)  [unwired: 1 in, 1 out]
        n229 = Select(t="EscribeTabla114", s=w525, f="Leer_Voltaje_4") -> (s? t:f=w523:string)
        n230 = call-poly "Enqueue Message.vi"("error in (no error)"=w528, "Message"=w523, "Message Queue"=w514) -> ("error out"=w526:errorcluster)  [unwired: 7 in, 1 out]
        n231 = call "Time Delay16"("error in (no error)"=w526, "Delay Time (s)"=1.0) -> ("error out"=w513:errorcluster)  [unwired: 9 in]
      }
      frame "EscribeTabla114" {
        # "col"
        n232 = call "FGV_fila.vi"("error in (no error)"=w536, "action"=enum16{"increment", "set_start", "get"}."get") -> ("error out"=w547:errorcluster, "fila out"=w542:i32)  [unwired: 2 in]
        n233 = Unbundle By Name(w532) -> ("Tabla"=w535:string[][])
        n234 = Unbundle By Name(w532) -> ("NPS"=w531:refnum<vi>)
        n235 = property class="DigNum (strict)"(reference=w531) -> ("Value"=w530:dbl)  [unwired: 1 in, 2 out]
        n236 = call "escribeEnTablaUnValor.vi"("element"=w530, "fila"=w542, "col"=2, "tabla in"=w535) -> ("tabla out"=w541:string[][])  [unwired: 7 in]
        n237 = local read "size_frec"() -> (w539:i32)
        n238 = call "FGV_fila.vi"("error in (no error)"=w547, "action"=enum16{"increment", "set_start", "get"}."increment") -> ("error out"=w546:errorcluster, "fila out"=w543:i32)  [unwired: 2 in]
        n239 = Bundle By Name(cluster=w532, "Tabla"=w541) -> (w540:refnum<class "AjustesPrevios.lvclass">)
        n240 = Greater Or Equal?(x=w543, y=w539) -> (x >= y?=w544:bool)
        n241 = case shown="True" w544 {
          tunnel: w546 -> [w550 w565]
          tunnel: [w555 w560] -> w545
          tunnel: w537 -> [w553 w559]
          tunnel: w533 -> [w551 w556]
          frame False {
            n242 = call "FGV_timer.vi"("error in (no error)"=w550, "time target"=w551, "action"=enum16{"get time", "start timer"}."start timer") -> ()  [unwired: 3 out]
            n243 = call-poly "Enqueue Message.vi"("error in (no error)"=w550, "Message"="Leer_Voltaje_4", "Message Queue"=w553) -> ("error out"=w555:errorcluster)  [unwired: 7 in, 1 out]
          }
          frame True {
            n244 = call "FGV_fila.vi"("fila_inicial"=0, "action"=enum16{"increment", "set_start", "get"}."set_start") -> ()  [unwired: 2 in, 2 out]
            n245 = One Button Dialog(message="Generación de frecuencias OK") -> ()  [unwired: 1 in, 1 out]
            n246 = local write "generar_CAM"(FALSE) -> ()
            n247 = call "FGV_timer.vi"("time target"=w556, "action"=enum16{"get time", "start timer"}."start timer") -> ()  [unwired: 1 in, 3 out]
            n248 = call-poly "Enqueue Message.vi"("error in (no error)"=w565, "Message"="detenerGEN", "Message Queue"=w559) -> ("error out"=w560:errorcluster)  [unwired: 7 in, 1 out]
          }
        }
        n249 = local read "Vguardado"() -> (w538:dbl)
        n250 = local write "voltaje"(w538) -> ()
      }
      frame "Exit" {
        w568 = TRUE
        # "#evangelio Manda a cerrar el EHL"
        # "#evangelio Manda a cerrar todos los Loops"
        n251 = Release Queue(queue=w572, error in (no error)=w573) -> (error out=w577:errorcluster)  [unwired: 1 in, 2 out]
        n252 = Unbundle By Name(w569) -> ("Control references"=w578:T7)
        n253 = for {
          tunnel: w567 -> [w581] mode=indexing
          tunnel: w570 -> [w580]
          tunnel: TRUE -> [w579]
          n254 = call-poly "Enqueue Message.vi"("Priority Message? (F)"=w579, "Message"=w580, "Message Queue"=w581) -> ()  [unwired: 7 in, 2 out]
        }
        n255 = call "Close All Ref.vi"("error in (no error)"=w577, "Control references"=w578) -> ("error out"=w575:errorcluster)  [unwired: 9 in]
        n256 = call "Fire User Event - Stop.vi"("error in (no error)"=w575, "Event Data"=w568, "User Event"="Exit EHL", "User Event in"=w571) -> ("error out"=w566:errorcluster)  [unwired: 7 in]
      }
      frame "Error" {
        n257 = Variant To Data(error in=w590, type=errorcluster {"status"=FALSE, "code"=0, "source"=""} ("error constant"), Variant=w589) -> (data=w591:errorcluster, error out=w588:errorcluster)
        n258 = call <vilib>:"Simple Error Handler.vi"("error in (no error)"=w591) -> ()  [unwired: 4 in, 5 out]
        n259 = call-poly "Enqueue Message.vi"("error in (no error)"=w588, "Message"="Detener_Instrumento", "Message Queue"=w586) -> ("error out"=w587:errorcluster, "dup Message Queue"=w583:refnum<queue>)  [unwired: 7 in]
        n260 = call-poly "Enqueue Message.vi"("error in (no error)"=w587, "Message"="Exit", "Message Queue"=w583) -> ("error out"=w584:errorcluster)  [unwired: 7 in, 1 out]
      }
      frame Default {
      }
      frame "--------------------------Controles---------------------------" {
      }
    }
    n261 = call "Error Handler - Event Handling Loop.vi"("error in (no error)"=w46, "Message Queue"=w45) -> ("dup error in"=w44:errorcluster)  [unwired: 7 in, 2 out]
    n262 = Unbundle By Name(w59) -> ("Tabla"=w58:string[][])
    n263 = local write "Tabla"(w58) -> ()
  }
  n264 = call "Inst_CNT90.vi"("error in"=w9, "All Message Queues in"=w13, "AjustesPrevios in"=w14) -> ()  [unwired: 8 in, 1 out]
  n265 = call "Inst_DS360.vi"("error in"=w9, "All Message Queues in"=w13, "AjustesPrevios in"=w14) -> ()  [unwired: 8 in, 1 out]
  n266 = call "Inst_K2002.vi"("error in"=w9, "All Message Queues in"=w13, "AjustesPrevios in"=w14) -> ()  [unwired: 8 in, 1 out]
  n267 = call "Inst_Nexus.vi"("error in"=w9, "All Message Queues in"=w13, "AjustesPrevios in"=w14) -> ()  [unwired: 8 in, 1 out]
  n268 = call "Inst_Pistofono.vi"("error in"=w9, "All Message Queues in"=w13, "AjustesPrevios in"=w14) -> ()  [unwired: 8 in, 1 out]
  n269 = while {
    tunnel: w16 -> [w600]
    shift-right: [w604] -> w24
    shift-left: w26 -> [w605]
    shift-right: [w601] -> w29
    shift-left: _ -> [_]
    stop <- w602 stop-if-true
    n270 = event shown="[6] \"generar\": Value Change" {
      selector: w605 -> [_ _ _ _ _ _ _ _ _ _ _ _ _]
      dyn-events: [_ _ _ _ _ _ _ _ _ _ _ _ _] -> w604
      timeout: _ -> [_ _ _ _ _ _ _ _ _ _ _ _ _]
      tunnel: w600 -> [w609 w611 w616 w626 w630 _ w643 w660 w665 w670 w680 _ w687]
      tunnel: [w608 _ w615 w622 w629 _ w641 w661 w667 w676 w681 w682 _] -> w603
      tunnel: [_ _ _ _ _ w634 _ _ _ _ _ _ _] -> w599
      tunnel: [_ _ _ _ _ _ _ _ _ _ _ _ w684] -> _
      event "Sensibilidad": Value Change {
        n271 = event-data() -> ()  [unwired: 1 in, 1 out]
        n272 = call-poly "Enqueue Message.vi"("Priority Message? (F)"=TRUE, "Message"="escribeSensib", "Message Queue"=w609) -> ("error out"=w608:errorcluster)  [unwired: 7 in, 1 out]
      }
      event Panel Close? {
        w610 = TRUE
        n273 = event-data() -> ()  [unwired: 1 in, 1 out]
        n274 = call-poly "Enqueue Message.vi"("Priority Message? (F)"=w610, "Message"="Confirmar Salida", "Message Queue"=w611) -> ()  [unwired: 7 in, 2 out]
        n275 = event-data("Discard?"=w610) -> ()  [unwired: 1 in, 1 out]
      }
      event "aplicar FC": Value Change {
        n276 = event-data() -> ()  [unwired: 1 in, 1 out]
        n277 = call-poly "Enqueue Message.vi"("Priority Message? (F)"=TRUE, "Message"="aplicarFC", "Message Queue"=w616) -> ("error out"=w615:errorcluster)  [unwired: 7 in, 1 out]
      }
      event "siguiente1": Value Change {
        n278 = event-data() -> ()  [unwired: 1 in, 1 out]
        n279 = Flush Queue(queue=w626) -> (queue out=w618:refnum<queue>, error out=w617:errorcluster)  [unwired: 1 in, 1 out]
        n280 = call-poly "Enqueue Message.vi"("Priority Message? (F)"=TRUE, "error in (no error)"=w617, "Message"="escribir_datos_igual_patrones", "Message Queue"=w618) -> ("error out"=w623:errorcluster, "dup Message Queue"=w624:refnum<queue>)  [unwired: 6 in]
        n281 = local write "voltaje a CAM"(0.0 ("NPS")) -> ()
        n282 = call-poly "Enqueue Message.vi"("error in (no error)"=w623, "Message"="preguntar_gen", "Message Queue"=w624) -> ("error out"=w622:errorcluster)  [unwired: 7 in, 1 out]
      }
      event "siguiente2": Value Change {
        n283 = event-data() -> ()  [unwired: 1 in, 1 out]
        n284 = Flush Queue(queue=w630) -> (queue out=w628:refnum<queue>, error out=w631:errorcluster)  [unwired: 1 in, 1 out]
        n285 = property on="Tabs" class="TabCtl (strict)"(error in=w631, "Value"=enum32{"Ajustes 1", "Ajustes 2", "Ajustes 3"}."Ajustes 3" ("Tabs")) -> (error out=w632:errorcluster)  [unwired: 1 in, 1 out]
        n286 = call-poly "Enqueue Message.vi"("error in (no error)"=w632, "Message"="AvisoPanelTrasero", "Message Queue"=w628) -> ("error out"=w629:errorcluster)  [unwired: 7 in, 1 out]
      }
      event User Event {
        n287 = event-data() -> ("User Event"=w636:string, "Event Data"=w635:variant)  [unwired: 1 in]
        n288 = case shown="\"Exit EHL\"" w636 {
          tunnel: w635 -> [_ w638]
          tunnel: [_ w637] -> w634
          frame Default {
          }
          frame "Exit EHL" {
            # "#evangelio Termina\nla ejecucion del EHL"
            n289 = Variant To Data(type=TRUE, Variant=w638) -> (data=w637:bool)  [unwired: 1 in, 1 out]
          }
        }
      }
      event "generar": Value Change {
        n290 = event-data() -> ("NewVal"=w640:bool)  [unwired: 1 in]
        n291 = Flush Queue(queue=w643) -> (queue out=w642:refnum<queue>, error out=w644:errorcluster)  [unwired: 1 in, 1 out]
        n292 = case shown="True" w640 {
          tunnel: w644 -> [w648 w657]
          tunnel: w642 -> [w649 w656]
          tunnel: [w647 w653] -> w641
          frame False {
            n293 = call-poly "Enqueue Message.vi"("Priority Message? (F)"=TRUE, "error in (no error)"=w648, "Message"="detenerGEN", "Message Queue"=w649) -> ("error out"=w647:errorcluster)  [unwired: 6 in, 1 out]
          }
          frame True {
            n294 = local read "ajusteAmp(mV)"() -> (w651:T1)
            n295 = call-poly "Enqueue Message.vi"("error in (no error)"=w657, "Message Data"=w651, "Message"="EnviarVoltajeGEN", "Message Queue"=w656) -> ("error out"=w654:errorcluster, "dup Message Queue"=w655:refnum<queue>)  [unwired: 6 in]
            n296 = call-poly "Enqueue Message.vi"("error in (no error)"=w654, "Message"="generar", "Message Queue"=w655) -> ("error out"=w653:errorcluster)  [unwired: 7 in, 1 out]
          }
        }
      }
      event Value Change {
        n297 = event-data() -> ()  [unwired: 1 in, 1 out]
        n298 = call-poly "Enqueue Message.vi"("Priority Message? (F)"=TRUE, "Message"="ModificarSeñal", "Message Queue"=w660) -> ("error out"=w661:errorcluster)  [unwired: 7 in, 1 out]
      }
      event "guardar": Value Change {
        n299 = event-data() -> ()  [unwired: 1 in, 1 out]
        n300 = Flush Queue(queue=w665) -> (queue out=w664:refnum<queue>, error out=w666:errorcluster)  [unwired: 1 in, 1 out]
        n301 = call-poly "Enqueue Message.vi"("Priority Message? (F)"=TRUE, "error in (no error)"=w666, "Message"="guardar", "Message Queue"=w664) -> ("error out"=w667:errorcluster)  [unwired: 6 in, 1 out]
      }
      event "anterior2": Value Change {
        n302 = event-data() -> ()  [unwired: 1 in, 1 out]
        n303 = property on="Tabs" class="TabCtl (strict)"("Value"=enum32{"Ajustes 1", "Ajustes 2", "Ajustes 3"}."Ajustes 1" ("Tabs")) -> (error out=w677:errorcluster)  [unwired: 2 in, 1 out]
        n304 = call-poly "Enqueue Message.vi"("error in (no error)"=w677, "Message"="detenerGEN", "Message Queue"=w670) -> ("error out"=w671:errorcluster, "dup Message Queue"=w669:refnum<queue>)  [unwired: 7 in]
        n305 = call-poly "Enqueue Message.vi"("error in (no error)"=w671, "Message"="reconec_pistofono", "Message Queue"=w669) -> ("error out"=w674:errorcluster, "dup Message Queue"=w673:refnum<queue>)  [unwired: 7 in]
        n306 = call-poly "Enqueue Message.vi"("error in (no error)"=w674, "Message"="Ajustes1", "Message Queue"=w673) -> ("error out"=w676:errorcluster)  [unwired: 7 in, 1 out]
      }
      event "terminar": Value Change {
        n307 = event-data() -> ()  [unwired: 1 in, 1 out]
        n308 = call-poly "Enqueue Message.vi"("Message"="Exit", "Message Queue"=w680) -> ("error out"=w681:errorcluster)  [unwired: 8 in, 1 out]
      }
      event "anterior3": Value Change {
        n309 = event-data() -> ()  [unwired: 1 in, 1 out]
        n310 = property on="Tabs" class="TabCtl (strict)"("Value"=enum32{"Ajustes 1", "Ajustes 2", "Ajustes 3"}."Ajustes 2" ("Tabs")) -> (error out=w682:errorcluster)  [unwired: 2 in, 1 out]
      }
      event "generar_CAM": Value Change {
        n311 = event-data() -> ()  [unwired: 1 in, 1 out]
        n312 = Flush Queue(queue=w687) -> (queue out=w686:refnum<queue>)  [unwired: 1 in, 2 out]
        n313 = call-poly "Enqueue Message.vi"("Message"="AvisoCAM_94", "Message Queue"=w686) -> ("error out"=w684:errorcluster)  [unwired: 8 in, 1 out]
      }
    }
    n314 = call "Error Handler - Event Handling Loop.vi"("error in (no error)"=w603, "Message Queue"=w600) -> ("dup error in"=w601:errorcluster, "Error?"=w598:bool)  [unwired: 7 in, 1 out]
    n315 = Or(x=w599, y=w598) -> (x .or. y?=w602:bool)
  }
  n316 = Unregister For Events(event registration refnum=w24, error in=w29) -> (error out=w25:errorcluster)
  n317 = disable-structure shown="Disabled" {
    disable-tunnel: w27 -> [w691 w693]
    disable-tunnel: [w690 w693] -> w23
    disable-tunnel: w11 -> [w689 w692]
    disable-tunnel: [w688 w692] -> w10
    frame Disabled {
      n318 = call-dynamic "CleanUp.vi"("error in (no error)"=w689, "AjustesPrevios in"=w691) -> ("error out"=w688:errorcluster, "AjustesPrevios out"=w690:refnum<class "AjustesPrevios.lvclass">)  [unwired: 8 in]
    }
    frame Enabled {
    }
  }
  "AjustesPrevios out" <- w23
  n319 = Merge Errors(w25, w10) -> (→"error out":errorcluster)
